vi "PI Open Interface.vi"(1 "Interface clear":string[](array[string])=["*idn?", "*idn?", "*idn?", "*idn?", "*idn?", "*idn?", "*idn?", "*idn?", "*idn?", "*idn?", "*idn?", "*idn?", "*idn?", "*idn?", "*idn?", "*idn?", "*idn?", "*idn?", "*idn?", "*idn?"], 2 "Number of systems":i32=1 min=1 step=1, 3 "Interface configuration":T10(array[cluster])=[{"RS232 Portnumber"=0, "Timeout"=5000, "RS232 Baud rate"=57600, "Interface"=0, "GPIB Bus"=0, "GPIB Address"=4, "GPIB Mode"=0}, {"RS232 Portnumber"=1, "Timeout"=5000, "RS232 Baud rate"=57600, "Interface"=0, "GPIB Bus"=0, "GPIB Address"=5, "GPIB Mode"=0}, {"RS232 Portnumber"=2, "Timeout"=5000, "RS232 Baud rate"=57600, "Interface"=0, "GPIB Bus"=0, "GPIB Address"=6, "GPIB Mode"=0}, {"RS232 Portnumber"=3, "Timeout"=5000, "RS232 Baud rate"=57600, "Interface"=0, "GPIB Bus"=0, "GPIB Address"=7, "GPIB Mode"=0}] {"Interface" items=["RS232", "GPIB", "DLL", "TCP-IP", "USB", "Analog"]; "RS232 Portnumber" items=["COM1", "COM2", "COM3", "COM4", "COM5", "COM6", "COM7", "COM8", "COM9", "COM10", "COM11", "COM12", "COM13", "COM14", "COM15", "COM16", "COM17", "COM18", "COM19", "COM20", "COM21", "COM22", "COM23", "COM24", "COM25", "COM26", "COM27", "COM28", "COM29", "COM30"]}, 4 "Strings to send":string[](array[string])=["*idn?", "*idn?", "*idn?", "*idn?", "*idn?", "*idn?", "*idn?", "*idn?", "*idn?", "*idn?", "*idn?", "*idn?", "*idn?", "*idn?", "*idn?", "*idn?", "*idn?", "*idn?", "*idn?", "*idn?"], 5 "error in":errorcluster, 6 "DLL Interface\nConfiguration":T8(array[cluster])=[{"DLL for Device"=0, "DLL Interface"=2, "Parameter"="1"}, {"DLL for Device"=0, "DLL Interface"=0, "Parameter"=""}, {"DLL for Device"=0, "DLL Interface"=1, "Parameter"=""}, {"DLL for Device"=0, "DLL Interface"=1, "Parameter"=""}] {"DLL for Device" items=["C-843", "C-844", "E-710", "C-843.PM", "C-865", "E-761", "Mercury", "E-755", "E-753", "C-866", "E-712", "E-725", "E-861", "C-867", "E-517", "E-816", "E-709", "PI_GCS2_DLL", "HydraPollux"]; "DLL Interface" items=["RS232", "GPIB", "Board", "TCP-IP", "USB", "RS232_DC", "USB_DC", "TCPIP_DC"]}, 7 "Bit settings and parity":T4(array[cluster])=[{"data bits"=8, "stop bits"=enum."1 bit", "parity"=enum."no parity"}, {"data bits"=8, "stop bits"=enum."1 bit", "parity"=enum."no parity"}, {"data bits"=8, "stop bits"=enum."1 bit", "parity"=enum."no parity"}, {"data bits"=8, "stop bits"=enum."1 bit", "parity"=enum."no parity"}] {"data bits" min=5 max=8 step=1}, 8 "TCP/IP\nConfiguration":T3(array[cluster])=[{"Host address/name"="localhost", "Port"=3000, "Board"=0}, {"Host address/name"="Z-A521-2.pi.ws", "Port"=3000, "Board"=0}, {"Host address/name"="Z-A521-2.pi.ws", "Port"=3000, "Board"=0}, {"Host address/name"="Z-A521-2.pi.ws", "Port"=3000, "Board"=0}], 9 "Flow control":T5(array[cluster])=[{"input XON/XOFF"=FALSE, "input HW Handshake"=FALSE, "input alt HW HShk"=FALSE, "output XON/XOFF"=FALSE, "output HW Handshake"=FALSE, "output alt HW HShk"=FALSE, "XOFF byte "=19, "XON byte"=17, "parity error byte"=0}, {"input XON/XOFF"=FALSE, "input HW Handshake"=FALSE, "input alt HW HShk"=FALSE, "output XON/XOFF"=FALSE, "output HW Handshake"=FALSE, "output alt HW HShk"=FALSE, "XOFF byte "=19, "XON byte"=17, "parity error byte"=0}, {"input XON/XOFF"=FALSE, "input HW Handshake"=FALSE, "input alt HW HShk"=FALSE, "output XON/XOFF"=FALSE, "output HW Handshake"=FALSE, "output alt HW HShk"=FALSE, "XOFF byte "=19, "XON byte"=17, "parity error byte"=0}, {"input XON/XOFF"=FALSE, "input HW Handshake"=FALSE, "input alt HW HShk"=FALSE, "output XON/XOFF"=FALSE, "output HW Handshake"=FALSE, "output alt HW HShk"=FALSE, "XOFF byte "=19, "XON byte"=17, "parity error byte"=0}] {"parity error byte" format="%.0x"; "XON byte" format="%.0x"; "XOFF byte" format="%.0x"}, 10 "Termination character":T2[](array[typedef])=[enum."LF", enum."LF", enum."LF", enum."LF"], 11 "Syntax":T1[](array[typedef])=[enum."GCS 1.0", enum."GCS 1.0", enum."GCS 1.0", enum."GCS 1.0", enum."GCS 1.0", enum."GCS 1.0", enum."GCS 1.0", enum."GCS 1.0", enum."GCS 1.0", enum."GCS 1.0", enum."GCS 1.0", enum."GCS 1.0", enum."GCS 1.0", enum."GCS 1.0", enum."GCS 1.0", enum."GCS 1.0", enum."GCS 1.0", enum."GCS 1.0", enum."GCS 1.0", enum."GCS 1.0"], 12 "Register DC":bool[](array[boolean])) -> (14 "String read":string[](array[string])=["\n"], 19 "error out":errorcluster)   [LabVIEW 2020]
doc: "Establishes communication with the connected systems. The interface and error statuses of all connected systems are cleared by this VI, which sends XXX (no command), *IDN? and ERR?. \n\nSee PI Open Interface of one system.vi for control settings."
uses:
  Available interfaces.ctl
  Available DLLs.ctl
  Available DLL interfaces.ctl
  Termination character.ctl
  Syntax.ctl
  Global1.vi
panel:
  out "DLL device ID's":i32[](array[numeric])
  # "This vi establishes communication with the connected systems. The interfaces and error statuses of all connected \nsystems are cleared by this vi, which sends XXX (no command), *IDN? and ERR?."
  # "Interface\nConfiguration"
  # "Other RS232 parameters:"
  # "TCP/IP:"
  # "DLL:"
  # "General:"
  # "RS232:"
  # "GPIB:"
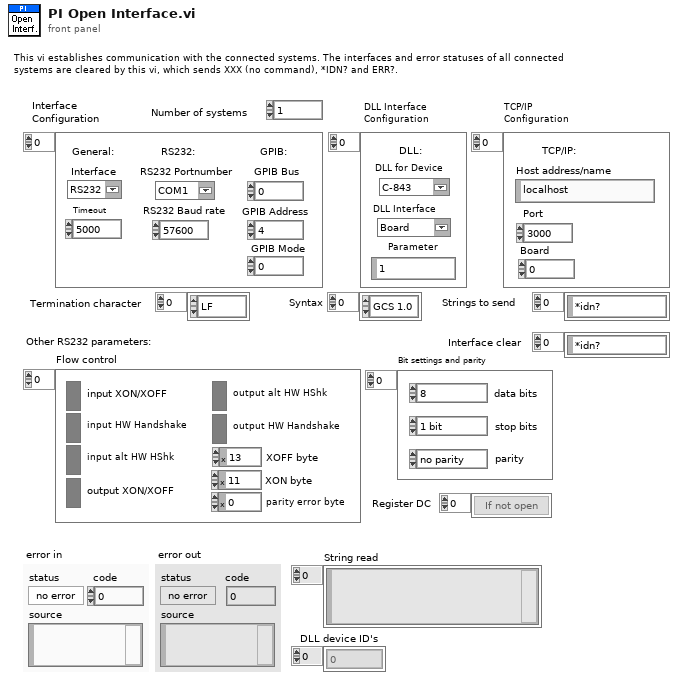
[diagram p1: front panel]
types:
  T1 = typedef "Syntax.ctl" = enum16{"GCS 1.0", "GCS 2.0", "GCS 3.0"}
  T2 = typedef "Termination character.ctl" = enum16{"LF", "CR", "LFCR", "CRLF"}
  T3 = cluster{"Host address/name":string, "Port":i32, "Board":i32}[]
  T4 = cluster{"data bits":u16, "stop bits":enum16{"1 bit", "1.5 bits", "2 bits"}, "parity":enum16{"no parity", "odd parity", "even parity", "mark parity", "space parity"}}[]
  T5 = cluster{"input XON/XOFF":bool, "input HW Handshake":bool, "input alt HW HShk":bool, "output XON/XOFF":bool, "output HW Handshake":bool, "output alt HW HShk":bool, "XOFF byte ":u8, "XON byte":u8, "parity error byte":u16}[]
  T6 = typedef "Available DLLs.ctl" = u16
  T7 = typedef "Available DLL interfaces.ctl" = u16
  T8 = cluster{"DLL for Device":T6, "DLL Interface":T7, "Parameter":string}[]
  T9 = typedef "Available interfaces.ctl" = u16
  T10 = cluster{"RS232 Portnumber":u16, "Timeout":u32, "RS232 Baud rate":u32, "Interface":T9, "GPIB Bus":i32, "GPIB Address":i32, "GPIB Mode":i32}[]
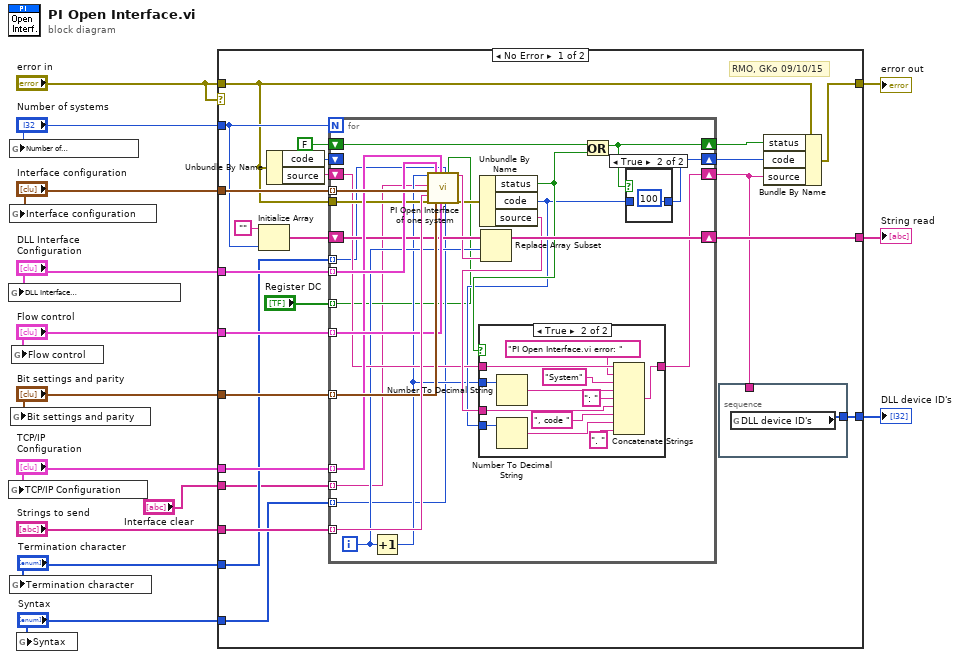
[diagram p0: block diagram]
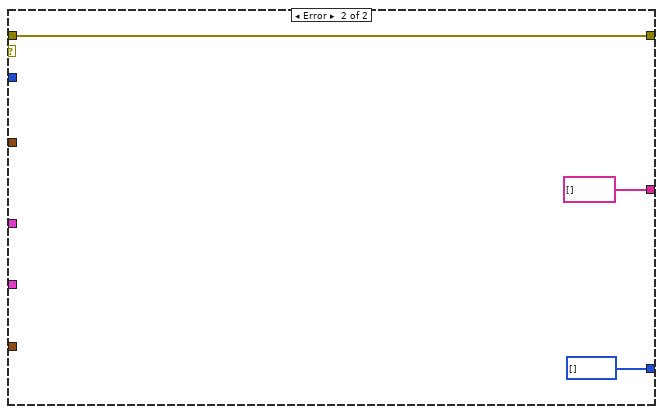
[diagram p4: hidden frame]
diagram:
  n1 = global write "Global1.vi" "DLL Interface\nConfiguration"("DLL Interface\nConfiguration") -> ()
  n2 = global write "Global1.vi" "TCP/IP Configuration"("TCP/IP\nConfiguration") -> ()
  n3 = global write "Global1.vi" "Number of\nsystems"("Number of systems") -> ()
  n4 = global write "Global1.vi" "Interface configuration"("Interface configuration") -> ()
  n5 = global write "Global1.vi" "Termination character"("Termination character") -> ()
  n6 = global write "Global1.vi" "Bit settings and parity"("Bit settings and parity") -> ()
  n7 = global write "Global1.vi" "Flow control"("Flow control") -> ()
  n8 = global write "Global1.vi" "Syntax"("Syntax") -> ()
  n9 = case shown="No Error" "error in" {
    tunnel: "DLL Interface\nConfiguration" -> [w37 _]
    tunnel: "Interface configuration" -> [w36 _]
    tunnel: "Number of systems" -> [w31 _]
    tunnel: "Flow control" -> [w35 _]
    tunnel: "Bit settings and parity" -> [w34 _]
    tunnel: "Strings to send" -> [w33 _]
    tunnel: "error in" -> [w21 w80]
    tunnel: "TCP/IP\nConfiguration" -> [w32 _]
    tunnel: [w27 string[] []] -> w6
    tunnel: [w26 w80] -> w5
    tunnel: [w23 i32[] [] ("DLL device ID's")] -> w4
    tunnel: "Termination character" -> [w18 _]
    tunnel: "Syntax" -> [w17 _]
    tunnel: "Interface clear" -> [w15 _]
    frame No Error {
      # "RMO, GKo 09/10/15"
      n10 = Initialize Array("", w31) -> (w29:string[])
      n11 = Unbundle By Name(w21) -> ("code"=w20:i32, "source"=w19:string)
      n12 = for {
        N: w31 -> [_]
        tunnel: w36 -> [w63] mode=indexing
        tunnel: w37 -> [w59] mode=indexing
        tunnel: w35 -> [w60] mode=indexing
        tunnel: w34 -> [w61] mode=indexing
        tunnel: w33 -> [w62] mode=indexing
        tunnel: w32 -> [w58] mode=indexing
        shift-right: [w55] -> w27
        shift-left: w29 -> [w57]
        shift-right: [w52] -> w25
        shift-left: FALSE -> [w47]
        shift-right: [w51] -> w24
        shift-left: w20 -> [_]
        shift-right: [w50] -> w22
        shift-left: w19 -> [w46]
        tunnel: w21 -> [w49]
        tunnel: w18 -> [w42] mode=indexing
        tunnel: w17 -> [w41] mode=indexing
        tunnel: "Register DC" -> [w40] mode=indexing
        tunnel: w15 -> [w39] mode=indexing
        i -> [w45]
        n13 = Increment(x=w45) -> (x+1=w43:i32)
        n14 = call "PI Open Interface of one system.vi"("System number"=w43, "Interface clear"=w39, "Interface configuration"=w63, "String to Send"=w62, "error in"=w49, "DLL Interface\nConfiguration"=w59, "Bit settings and parity"=w61, "TCP/IP\nConfiguration"=w58, "Flow control"=w60, "Termination character"=w42, "Syntax"=w41, "Register DC"=w40) -> ("String read"=w56:string, "error out"=w54:errorcluster)  [unwired: 6 out]
        n15 = Unbundle By Name(w54) -> ("status"=w48:bool, "code"=w44:i32, "source"=w53:string)
        n16 = case shown="True" w48 {
          tunnel: w46 -> [w64 w76]
          tunnel: w53 -> [_ w73]
          tunnel: [w64 w71] -> w50
          tunnel: w43 -> [_ w69]
          tunnel: w44 -> [_ w67]
          frame False {
          }
          frame True {
            n17 = Number To Decimal String(number=w69) -> (decimal integer string=w70:string)  [unwired: 1 out]
            n18 = Number To Decimal String(number=w67) -> (decimal integer string=w68:string)  [unwired: 1 out]
            n19 = Concatenate Strings(w76, "PI Open Interface.vi error: " ("string"), "System" ("string"), w70, ": " ("string"), w73, ", code " ("string"), w68, ". " ("string")) -> (w71:string)
          }
        }
        n20 = Replace Array Subset(array=w57, new element=w56, index=w45) -> (w55:string[])
        n21 = Or(x=w47, y=w48) -> (x .or. y?=w52:bool)
        n22 = case shown="True" w52 {
          tunnel: [w77 100 ("code")] -> w51
          tunnel: w44 -> [w77 _]
          frame False {
          }
          frame True {
          }
        }
      }
      n23 = stacked-sequence {
        tunnel: [w38] -> w23
        tunnel: w22 -> [_]
        frame #0 {
          n24 = global read "Global1.vi" "DLL device ID's"() -> (w38:i32[])
        }
      }
      n25 = Bundle By Name(cluster=w21, "status"=w25, "code"=w24, "source"=w22) -> (w26:errorcluster)
    }
    frame Error {
    }
  }
  "error out" <- w5
  "String read" <- w6
  "DLL device ID's" <- w4
